vi "OAT Sampled Power Spectrum.vi"   [LabVIEW 2017]
doc: "Computes the single-sided, scaled auto power spectrum of a time-domain signal. You can define the number of frequency bins."
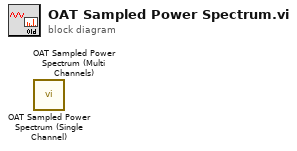
[diagram p0: block diagram]
diagram:
  n1 = call <vilib>:"OAT Sampled Power Spectrum (Single Channel).vi"() -> ()  [unwired: 9 in, 3 out]
  n2 = call <vilib>:"OAT Sampled Power Spectrum (Multi Channels).vi"() -> ()  [unwired: 9 in, 3 out]
